vi "Single test point on oscilliscope.vi"(11 "VISA resource name":refnum<visa-resource-name>="USB0::0x1AB1::0x0488::DS1BA202100064::INSTR") -> ()   [LabVIEW 2018]
uses:
  <instrlib>/RIGOL DS1000 Series/Public/Data/Read (Single Waveform).vi
  <instrlib>/RIGOL DS1000 Series/RIGOL DS1000 Series.lvlib
panel:
  out "RMS":dbl
  out "Mean (DC)":dbl
  out "Waveform Data":waveform(dbl)(graph)
  out "Numeric":i32
  out "Frequency":dbl
  out "Duty Cycle":dbl
  out "Period 2":dbl
  in  "Channel (0: Channel 1)":u16(ring) items=["Channel 1", "Channel 2", "Channel 3", "Channel 4"]
  in  "Stop":bool
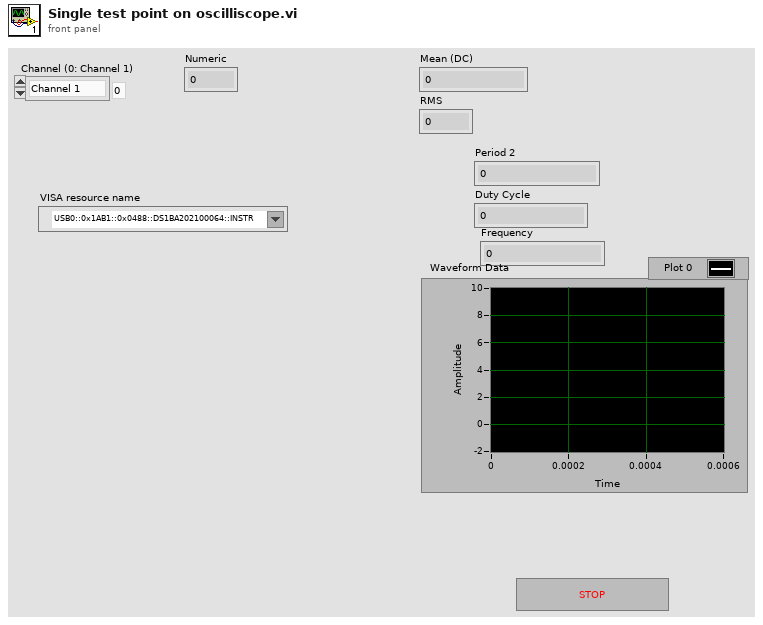
[diagram p1: front panel]
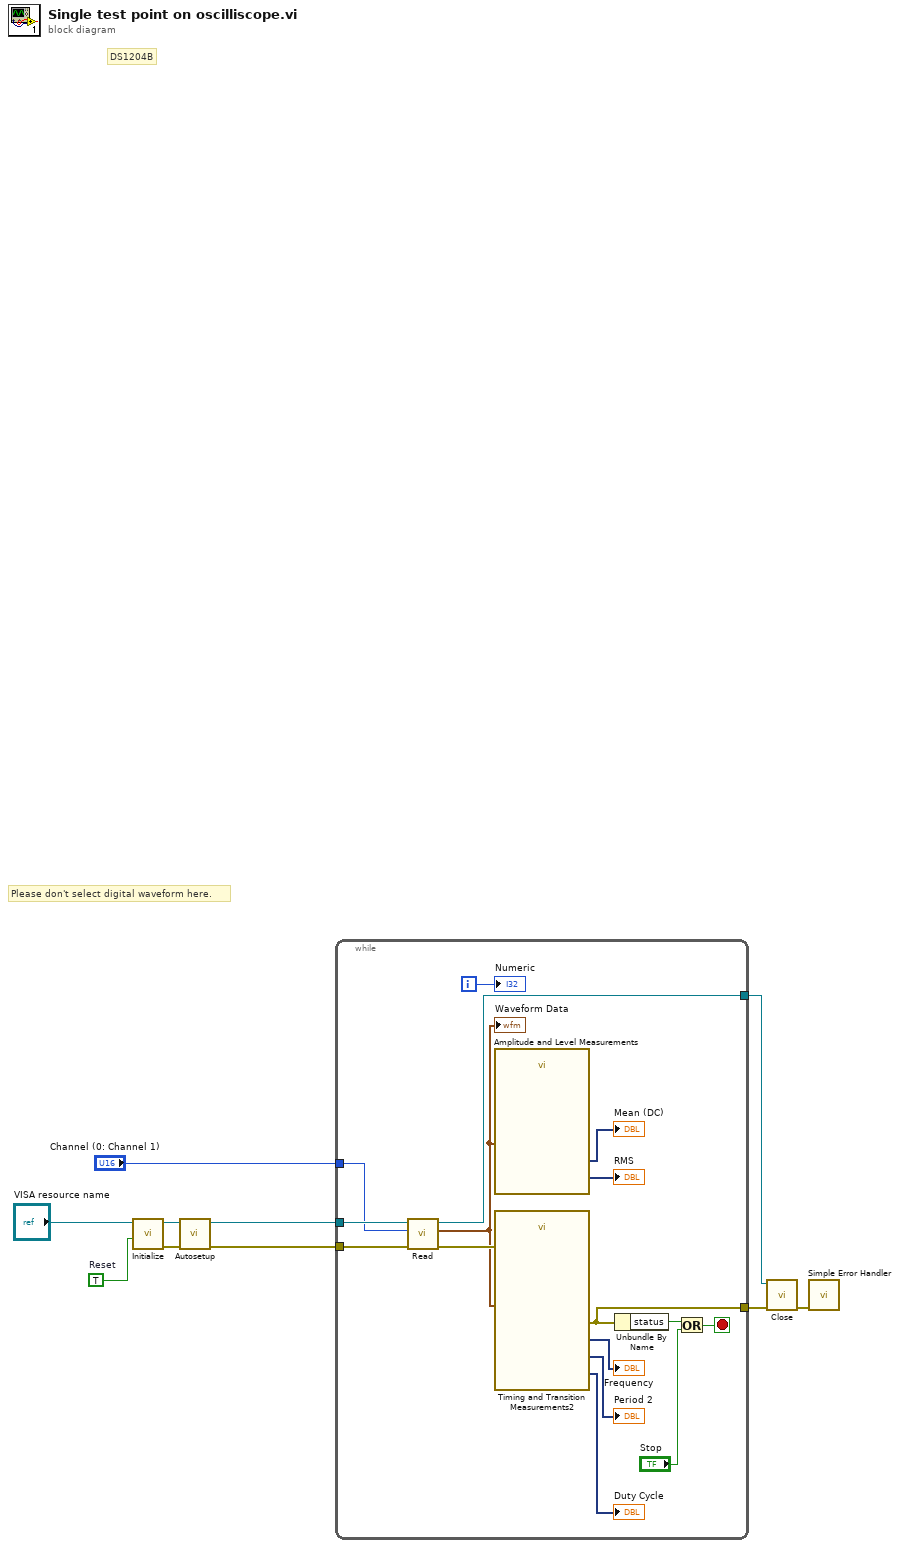
[diagram p0: block diagram]
diagram:
  w8 = TRUE  # Reset
  # "DS1204B"
  # "Please don't select digital waveform here."
  n1 = call <instrlib>:"Initialize.vi"("Reset (True)"=w8, "VISA resource name"="VISA resource name") -> ("error out"=w6:errorcluster, "VISA resource name out"=w7:refnum<visa-resource-name>)  [unwired: 2 in, 6 out]
  n2 = call <instrlib>:"Autosetup.vi"("error in (no error)"=w6, "VISA resource name"=w7) -> ("error out"=w9:errorcluster, "VISA resource name out"=w10:refnum<visa-resource-name>)  [unwired: 8 in]
  n3 = while {
    tunnel: w10 -> [w26]
    tunnel: w9 -> [w25]
    tunnel: "Channel (0: Channel 1)" -> [w18]
    tunnel: [w22] -> w2
    tunnel: [w19] -> w1
    i -> [w17]
    stop <- w24 stop-if-true
    n4 = call-poly <instrlib>:"Read.vi"("error in (no error)"=w25, "Channel (0: Channel 1)"=w18, "VISA resource name"=w26) -> ("error out"=w20:errorcluster, "Waveform Data"=w16:waveform(dbl), "VISA resource name out"=w22:refnum<visa-resource-name>)  [unwired: 6 in]
    "Waveform Data" <- w16
    n5 = call "Amplitude and Level Measurements"("Signals"=w16) -> ("Mean (DC)"=→"Mean (DC)":dynamicdata, "RMS"=→"RMS":dynamicdata)  [unwired: 12 in, 1 out]
    n6 = call "Timing and Transition Measurements2"("error in (no error)"=w20, "Signals"=w16) -> ("error out"=w19:errorcluster, "Frequency"=→"Frequency":dynamicdata, "Period"=→"Period 2":dynamicdata, "Duty Cycle"=→"Duty Cycle":dynamicdata)  [unwired: 6 in]
    n7 = Unbundle By Name(w19) -> ("status"=w21:bool)
    n8 = Or(x=w21, y="Stop") -> (x .or. y?=w24:bool)
    "Numeric" <- w17
  }
  n9 = call <instrlib>:"Close.vi"("error in (no error)"=w1, "VISA resource name"=w2) -> ("error out"=w3:errorcluster)  [unwired: 9 in]
  n10 = call <vilib>:"Simple Error Handler.vi"("error in (no error)"=w3) -> ()  [unwired: 1 in, 8 out]
